vi "Visualize nodes.vi"(1 "Max number (for centering)":i8, 2 "X 2":i8, 3 "Nodes 2":i8, 4 "X 1":i8, 5 "Nodes 1":i8) -> (0 "XY Graph":cluster{dbl[], dbl[]}[](array[cluster]) {"?" format="%.2f"; "?" format="%.2f"})   [LabVIEW 2010]
doc: "This VI generates to numbers (coordinates) for single layer of nodes (neurons). It is used for display purposes only."
panel:
  out "XY Graph 2":cluster{dbl[], dbl[]}[](graph)
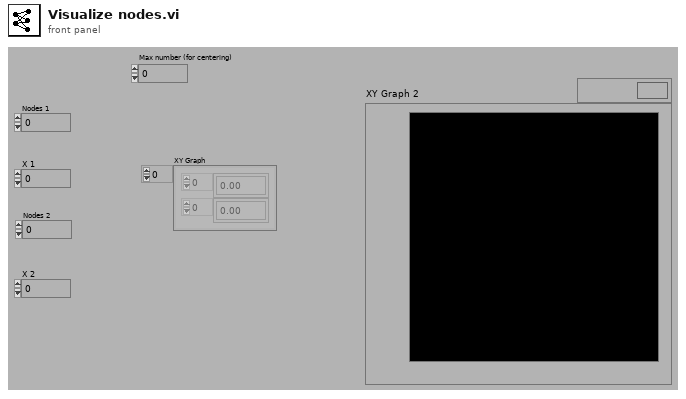
[diagram p1: front panel]
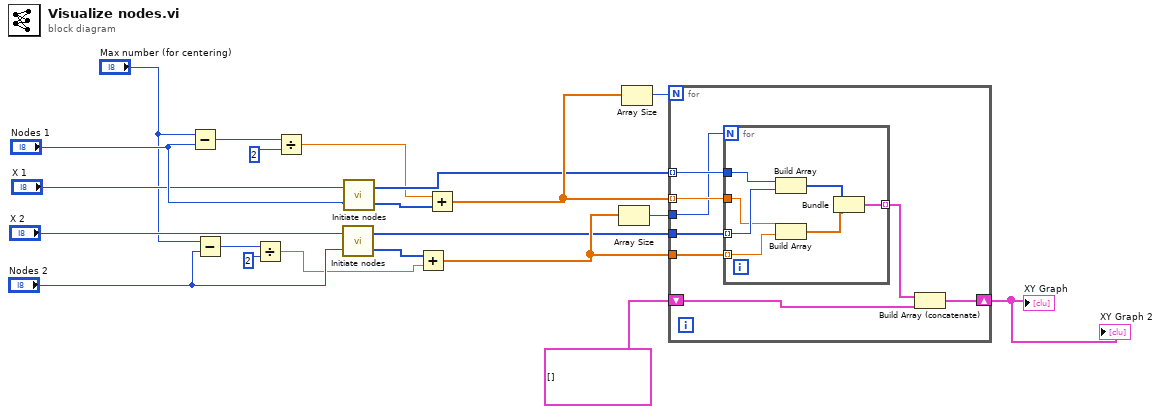
[diagram p0: block diagram]
diagram:
  n1 = Subtract(x="Max number (for centering)", y="Nodes 1") -> (x-y=w18:i8)
  n2 = Subtract(x="Max number (for centering)", y="Nodes 2") -> (x-y=w14:i8)
  n3 = Divide(x=w14, y=2) -> (x/y=w2:dbl)
  n4 = Divide(x=w18, y=2) -> (x/y=w3:dbl)
  n5 = call "Initiate nodes.vi"("Inputs"="Nodes 2", "X"="X 2") -> ("Y"=w7:i8[], "X"=w12:i8[])
  n6 = call "Initiate nodes.vi"("Inputs"="Nodes 1", "X"="X 1") -> ("Y"=w6:i8[], "X"=w11:i8[])
  n7 = Add(x=w7, y=w2) -> (x+y=w16:dbl[])
  n8 = Add(x=w3, y=w6) -> (x+y=w19:dbl[])
  n9 = Array Size(array=w16) -> (size(s)=w8:i32)
  n10 = Array Size(array=w19) -> (size(s)=w5:i32)
  n11 = for {
    N: w5 -> [_]
    tunnel: w11 -> [w29] mode=indexing
    tunnel: w19 -> [w28] mode=indexing
    tunnel: w12 -> [w27]
    tunnel: w16 -> [w26]
    shift-right: [w23] -> w1
    shift-left: cluster{dbl[], dbl[]}[] [] -> [w24]
    tunnel: w8 -> [w22]
    n12 = for {
      N: w22 -> [_]
      tunnel: w29 -> [w36]
      tunnel: w28 -> [w34]
      tunnel: w27 -> [w35] mode=indexing
      tunnel: w26 -> [w33] mode=indexing
      tunnel: [w30] -> w25 mode=indexing
      n13 = Build Array(w36, w35) -> (w32:i8[])
      n14 = Build Array(w34, w33) -> (w31:dbl[])
      n15 = Bundle(w32, w31) -> (w30:cluster{i8[], dbl[]})  [unwired: 1 in]
    }
    n16 = Build Array (concatenate)(w25, w24) -> (w23:cluster{dbl[], dbl[]}[])
  }
  "XY Graph" <- w1
  "XY Graph 2" <- w1
